vi "Set Front Panel State.vi"(8 "error in (no error)":errorcluster, 9 "Front Panel Window:State":T1(ring), 10 "View Hierarchy Level":i32, 11 "GUI View in":refnum<class "GUI View.lvclass">) -> (0 "error out":errorcluster, 3 "GUI View out":refnum<class "GUI View.lvclass">)   [LabVIEW 2023, in "GUI Views.lvlib" / "GUI View.lvclass"]
doc: "Sets the state of the Front Panel of a specified Actor Core VI of the the specified View class hierarchy. The method is active only if the GUI View is not contained. The Front Panel is specified by: \n\n<b> View Hierarchy Level</b> the level on the subclassing hierarchy of the GUI View actor, it is used to choose the Actor Core Front Panel among all the exisiting sublcasses of the GUI VIew Actor present in the View specified above"
uses:
  GUI View.lvclass
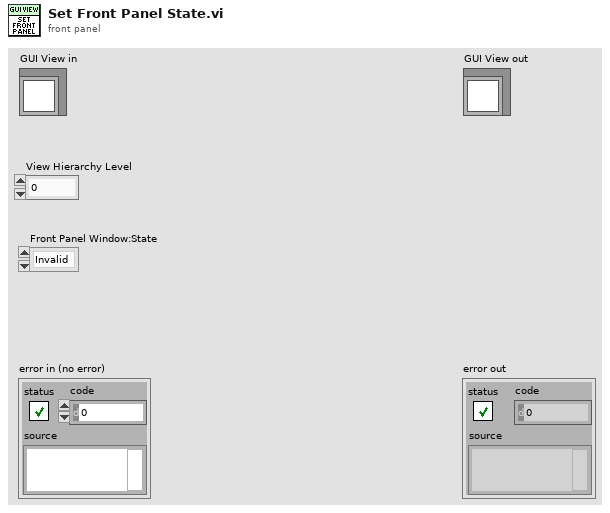
[diagram p1: front panel]
types:
  T1 = enum32{"Invalid", "Standard", "Closed", "Hidden", "Minimized", "Maximized"}
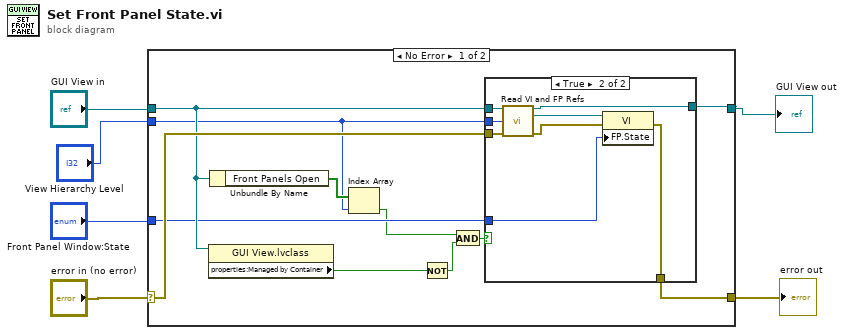
[diagram p0: block diagram]
diagram:
  n1 = case shown="No Error" "error in (no error)" {
    selector: "error in (no error)" -> [w17 w29]
    tunnel: [w15 w29] -> w2
    tunnel: [w16 w28] -> w1
    tunnel: "GUI View in" -> [w13 w28]
    tunnel: "Front Panel Window:State" -> [w11 _]
    tunnel: "View Hierarchy Level" -> [w7 _]
    frame No Error {
      n2 = property class="GUI View.lvclass"(reference=w13) -> ("properties:Managed by Container"=w14:bool)  [unwired: 1 in, 2 out]
      n3 = Unbundle By Name(w13) -> ("Front Panels Open"=w12:bool[])
      n4 = Index Array(array=w12, index=w7) -> (element=w9:bool)
      n5 = Not(x=w14) -> (.not. x?=w10:bool)
      n6 = And(x=w9, y=w10) -> (x .and. y?=w8:bool)
      n7 = case shown="True" w8 {
        tunnel: w11 -> [_ w26]
        tunnel: w17 -> [w18 w25]
        tunnel: w7 -> [_ w23]
        tunnel: [w19 w22] -> w16
        tunnel: [w18 w21] -> w15
        tunnel: w13 -> [w19 w20]
        frame False {
        }
        frame True {
          n8 = call "Read VI and FP Refs.vi"("GUI View in"=w20, "View Hierarchy Level"=w23, "error in (no error)"=w25) -> ("GUI View out"=w22:refnum<class "GUI View.lvclass">, "VI Ref"=w27:refnum<vi>, "error out"=w24:errorcluster)  [unwired: 8 in, 2 out]
          n9 = property class="VI"(reference=w27, error in=w24, "FP.State"=w26) -> (error out=w21:errorcluster)  [unwired: 1 out]
        }
      }
    }
    frame Error {
    }
  }
  "error out" <- w2
  "GUI View out" <- w1
